vi "Generate BER Curve Raw.vi"(4 "M-PSK":i32=16, 6 "Sample Step":dbl=1.0, 7 "Samples":i32=30, 9 "Message Bits":i32=500, 10 "Synchronization Sequence":i32=40, 11 "Zero Pad":i32=40) -> (0 "error out":errorcluster, 3 "BER Curve":dbl[](array[numeric]))   [LabVIEW 2013]
panel:
  out "Current Value":dbl
  in  "Averaging Number":i32=100
  out "Waveform Graph":dbl[](graph)
  in  "Initial Value":i32
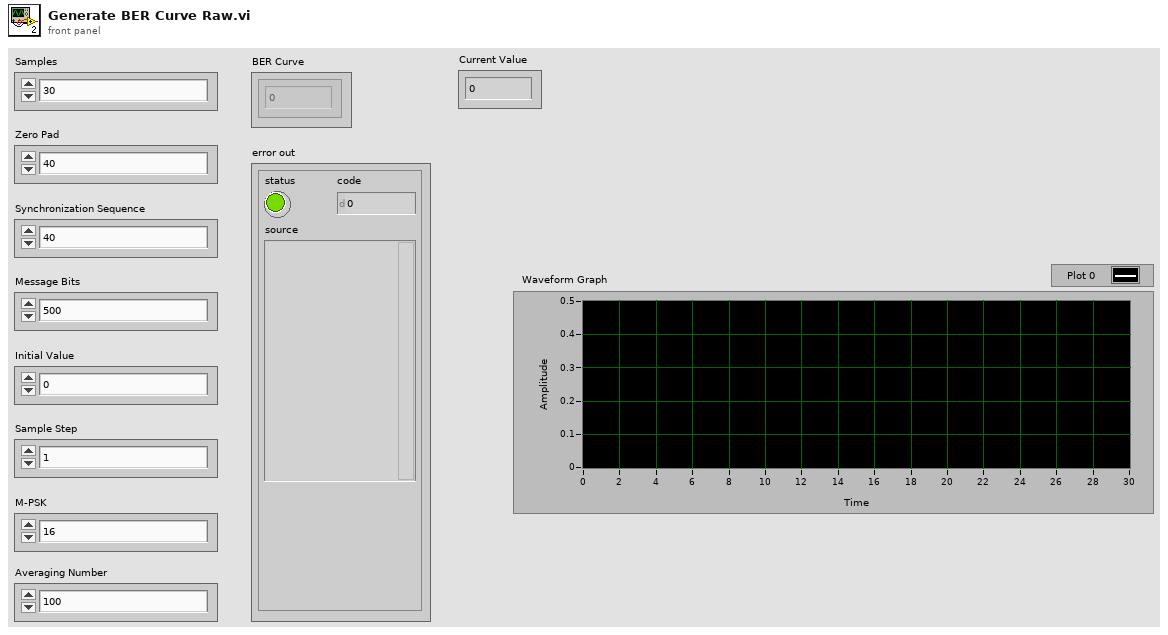
[diagram p1: front panel]
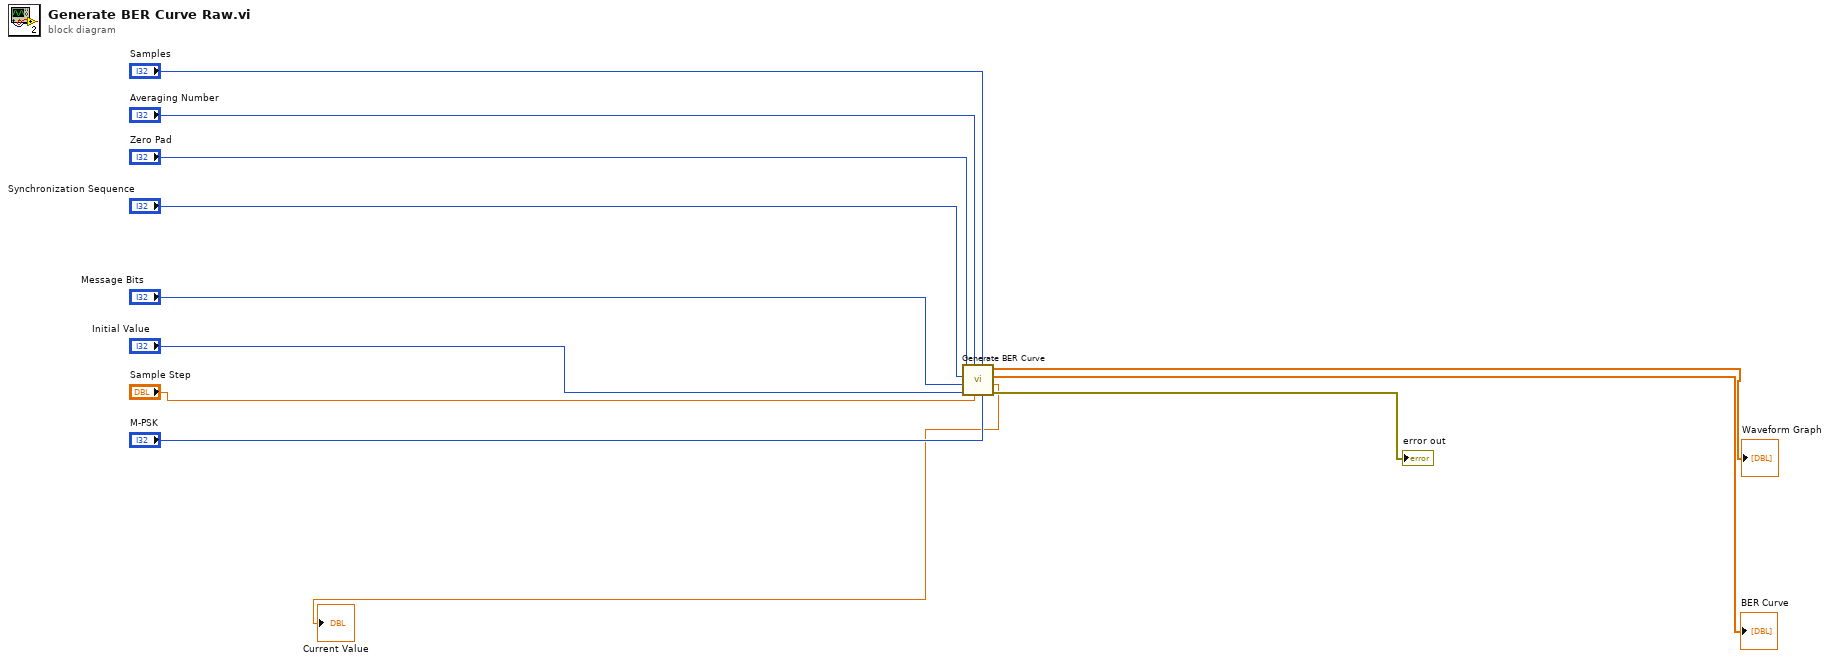
[diagram p0: block diagram]
diagram:
  n1 = call "Generate BER Curve.vi"("M-PSK"="M-PSK", "Samples"="Samples", "Sample Step"="Sample Step", "Averaging Number"="Averaging Number", "Initial Value"="Initial Value", "Message Bits"="Message Bits", "Synchronization Sequence"="Synchronization Sequence", "Zero Pad"="Zero Pad") -> ("error out"=→"error out":errorcluster, "Current Value"=→"Current Value":dbl, "BER Curve"=→"BER Curve":dbl[], "Waveform Graph"=→"Waveform Graph":dbl[])
